vi "SetGXMLCfgThrmcpl.vi"(8 "error in (no error)":errorcluster, 10 "ThrmcplChanCfg":T1, 11 "Thermocouple in":refnum<class "Thermocouple.lvclass">) -> (0 "error out":errorcluster, 3 "Thermocouple out":refnum<class "Thermocouple.lvclass">)   [LabVIEW 2018, in "Measurement Channels.lvlib" / "Thermocouple.lvclass"]
uses:
  Thermocouple.lvclass
  ThrmcplProps_TD.ctl
  Thermocouple.lvclass/Thermocouple.ctl
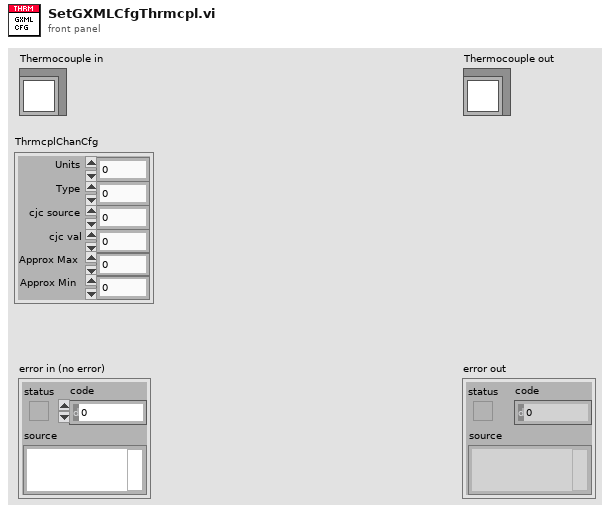
[diagram p1: front panel]
types:
  T1 = typedef "Measurement Channels.lvlib/Thermocouple.lvclass/ThrmcplProps_TD.ctl" = cluster{"Units":u16, "Type":u16, "cjc source":u16, "cjc val":dbl, "Approx Max":dbl, "Approx Min":dbl}
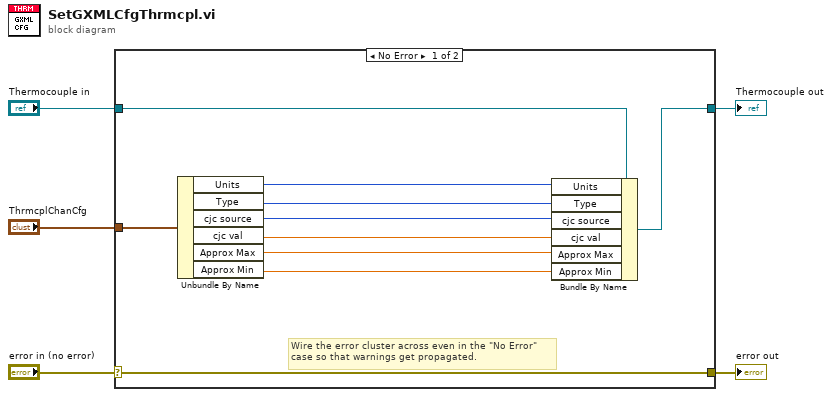
[diagram p0: block diagram]
diagram:
  n1 = case shown="No Error" "error in (no error)" {
    selector: "error in (no error)" -> [w15 w17]
    tunnel: [w15 w17] -> w4
    tunnel: [w6 w16] -> w2
    tunnel: "Thermocouple in" -> [w7 w16]
    tunnel: "ThrmcplChanCfg" -> [w8 _]
    frame No Error {
      # "Wire the error cluster across even in the \"No Error\"\ncase so that warnings get propagated."
      n2 = Unbundle By Name(w8) -> ("Units"=w14:u16, "Type"=w13:u16, "cjc source"=w12:u16, "cjc val"=w11:dbl, "Approx Max"=w10:dbl, "Approx Min"=w9:dbl)
      n3 = Bundle By Name(cluster=w7, "Units"=w14, "Type"=w13, "cjc source"=w12, "cjc val"=w11, "Approx Max"=w10, "Approx Min"=w9) -> (w6:refnum<class "Thermocouple.lvclass">)
    }
    frame Error {
    }
  }
  "error out" <- w4
  "Thermocouple out" <- w2
